vi "API Send Authorized Commands.vi"(7 "Commands":T1[](array[typedef]), 8 "error in (no error)":errorcluster, 9 "Timeout ms (5000)":i32=5000) -> (0 "error out":errorcluster, 1 "Timed Out?":bool, 5 "Responses":T2[](array[typedef]))   [LabVIEW 2011]
uses:
  Controls/PIM.API.Response.Unique.ctl
  Controls/PIM.API.Response.Samples.ctl
  iQA Sweep Behavior.ctl
  Controls/PIM.API.Command.Unique.ctl
  HWIO Global.vi
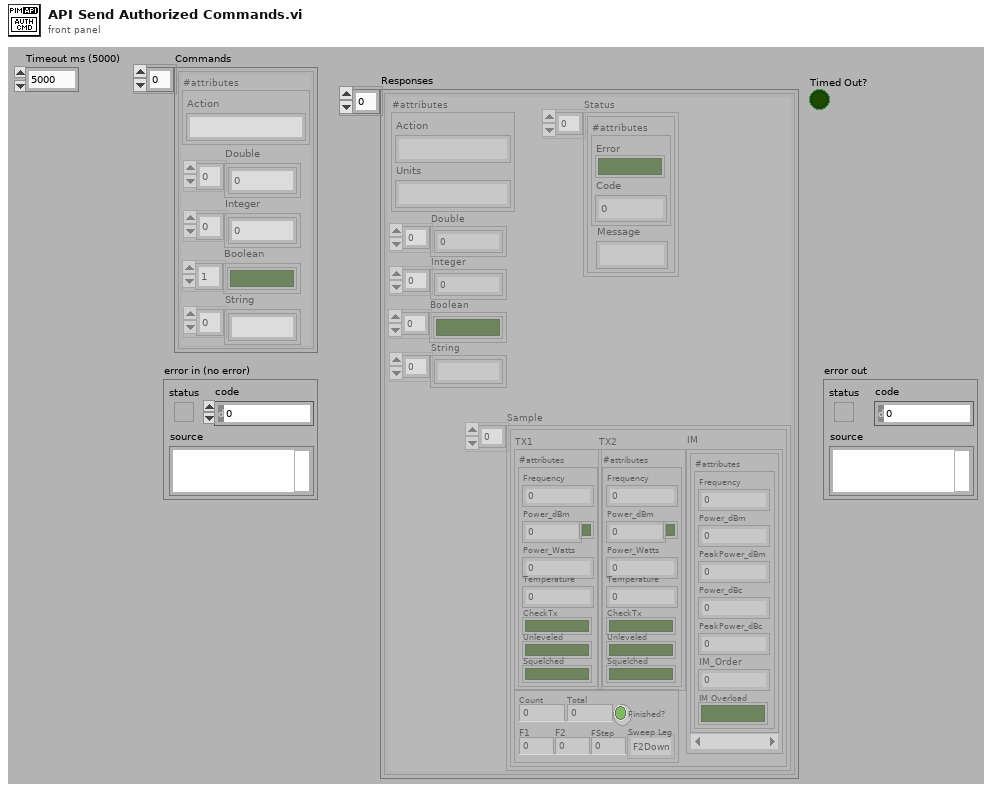
[diagram p1: front panel]
types:
  T1 = typedef "PIM.API.Command.Unique.ctl" = cluster{"#attributes":cluster{"Action":string}, "Double":dbl[], "Integer":i32[], "Boolean":bool[], "String":string[]}
  T2 = typedef "PIM.API.Response.Unique.ctl" = cluster{"#attributes":cluster{"Action":string, "Units":string}, "Double":dbl[], "Integer":i32[], "Boolean":bool[], "String":string[], "Sample":T3[], "Status":cluster{"#attributes":cluster{"Error":bool, "Code":i32}, "Message":string}[]}
  T3 = typedef "PIM.API.Response.Samples.ctl" = cluster{"TX1":cluster{"#attributes":cluster{"Frequency":dbl, "Power_dBm":dbl, "Power_Watts":dbl, "CheckTx":bool, "Unleveled":bool, "Squelched":bool, "Temperature":dbl, "ToneOn":bool}}, "TX2":cluster{"#attributes":cluster{"Frequency":dbl, "Power_dBm":dbl, "Power_Watts":dbl, "CheckTx":bool, "Unleveled":bool, "Squelched":bool, "Temperature":dbl, "ToneOn":bool}}, "IM":cluster{"#attributes":cluster{"Frequency":dbl, "Power_dBm":dbl, "PeakPower_dBm":dbl, "Power_dBc":dbl, "PeakPower_dBc":dbl, "IM_Order":u8, "IM Overload":bool}}[], "#attributes":cluster{"Count":u32, "Total":u32, "Finished?":bool, "Sweep Leg":T4, "F1":dbl, "F2":dbl, "FStep":dbl}}
  T4 = typedef "iQA Sweep Behavior.ctl" = enum16{"F2Down", "F1Up", "RxMultiIM"}
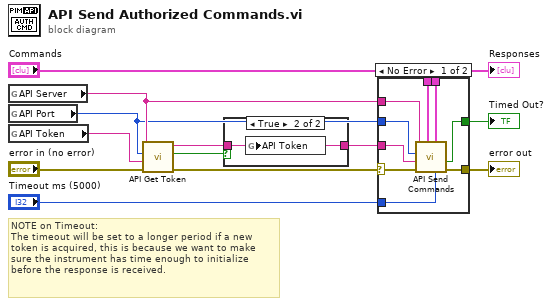
[diagram p0: block diagram]
diagram:
  # "NOTE on Timeout: \nThe timeout will be set to a longer period if a new token is acquired, this is because we want to make sure the instrument has time enough to initialize before the response is received."
  n1 = global read "HWIO Global.vi" "API Server"() -> (w9:string)
  n2 = global read "HWIO Global.vi" "API Port"() -> (w8:u16)
  n3 = global read "HWIO Global.vi" "API Token"() -> (w5:string)
  n4 = call "API Get Token.vi"("error in (no error)"="error in (no error)", "Existing Token"=w5, "API Port (80)"=w8, "API Server (localhost)"=w9) -> ("error out"=w7:errorcluster, "New token retrieved?"=w4:bool, "Token"=w3:string)  [unwired: 5 in]
  n5 = case shown="True" w4 {
    tunnel: w3 -> [w14 w15]
    tunnel: [w14 w15] -> w2
    frame False {
    }
    frame True {
      n6 = global write "HWIO Global.vi" "API Token"(w15) -> ()
    }
  }
  n7 = case shown="No Error" w7 {
    selector: w7 -> [w18 w25]
    tunnel: w2 -> [w24 _]
    tunnel: [w23 _] -> w12
    tunnel: "Commands" -> [w22 _]
    tunnel: [w21 w25] -> w10
    tunnel: w9 -> [w20 _]
    tunnel: w8 -> [w19 _]
    tunnel: "Timeout ms (5000)" -> [w17 _]
    tunnel: [w16 _] -> w1
    frame No Error {
      n8 = call "API Send Commands.vi"("Timeout ms (30000)"=w17, "Commands"=w22, "error in (no error)"=w18, "Token"=w24, "API Port (80)"=w19, "API Server (localhost)"=w20) -> ("error out"=w21:errorcluster, "Timed Out?"=w16:bool, "Responses"=w23:T2[])  [unwired: 2 in, 1 out]
    }
    frame Error {
    }
  }
  "Responses" <- w12
  "error out" <- w10
  "Timed Out?" <- w1
